vi "Hardware - NI 9751-3 (DI Driver) Host.vi"() -> ()   [LabVIEW 2015, in "ECS-Host.lvlib"]
uses:
  ECS-Host.lvlib
  <vilib>/addons/Software Calibration Management/XControls/SubHost.xctl
panel:
  in  "DisableOnCrit":bool caption="Disable On Crit?"
  in  "OpenCircuitOverride":bool
  in  "Clear Faults":bool
  out "FPGAReadError":bool
  out "FPGAWriteError":bool
  in  "OneShot":bool
  out "ShortCircuitFault":bool
  out "PSOverloadFault":bool
  out "PSChargeFault":bool
  out "ModuleTempFault":bool
  out "LowVoltageDriverFault":bool
  out "HighVoltageLimitFault":bool
  out "HighVoltageDriverFault":bool
  out "FI3OpenCircuit":bool
  out "FI2OpenCircuit":bool
  out "FI1OpenCircuit":bool
  out "Ch3TimingViolation":bool
  out "Ch3PulseOverlap":bool
  out "Ch2TimingViolation":bool
  out "Ch2PulseOverlap":bool
  out "Ch1TimingViolation":bool
  out "Ch1PulseOverlap":bool
  out "MinOffTimeCAD":sgl caption="[]"
  in  "MinOffTime":sgl caption="[]"
  in  "Ch3Enable":bool
  in  "ModuleEnable":bool
  in  "InjectionEnable":bool
  in  "PowerSupplyEnable":bool
  out "ModulePresent":bool
  in  "Phase1FirstPeakEnable":bool
  in  "PiezoEnable":bool
  in  "PiezoInvert":bool
  in  "OneShotSelect":enum32{"a", "b", "c", "d"}(ring)
  in  "OneShotTime":sgl caption="[msec]" format="%#.3f"
  in  "DI3 Scope":T1(xcontrol)
  in  "_DI3_IPhaseDriveArray":bool[](array[boolean]) caption="IPhaseDriveArray"
  in  "IPhaseDuration":sgl[](array[numeric]) min=0 max=5 step=0.001 format="%#.3g"
  in  "IPhaseCurrentLower":sgl[](array[numeric]) min=0 max=30 step=0.1 format="%#.3g"
  in  "IPhaseCurrentUpper":sgl[](array[numeric]) min=0 max=30 step=0.1 format="%#.3g"
  out "BatteryVoltage":sgl=21.08 caption="Battery Voltage"
  out "InternalHighVoltage":sgl=100.0 caption="Internal High Voltage" max=100
  out "ExternalHighVoltage":sgl caption="External High Voltage"
  out "_OLIntegrator_Display":sgl caption="Overload Integrator" format="%#.1g"
  out "ModuleTemperature":sgl=21.08 caption="Module Temp"
  in  "BackBoostTime":sgl caption="[msec]" min=0 max=0.4 step=0.01 format="%#.3f"
  in  "HighVTarget":sgl caption="[V]" max=100 format="%#.1f"
  out "ModuleRev":string
  in  "Ch2Enable":bool
  in  "Ch1Enable":bool
  out "OLIntegrator":u32 caption="Overload Integrator"
  in  "IPhaseDrive":u8
  # "[C]"
  # "Module Temp"
  # "Battery Voltage"
  # "[V]"
  # "Internal High Voltage"
  # "[V]"
  # "External High Voltage"
  # "[V]"
  # "Overload Integrator"
  # "[%]"
  # "[Amps]"
  # "[Amps]"
  # "[ms]"
  # "1"
  # "2"
  # "3"
  # "4"
  # "5"
  # "6"
  # "7"
  # "8"
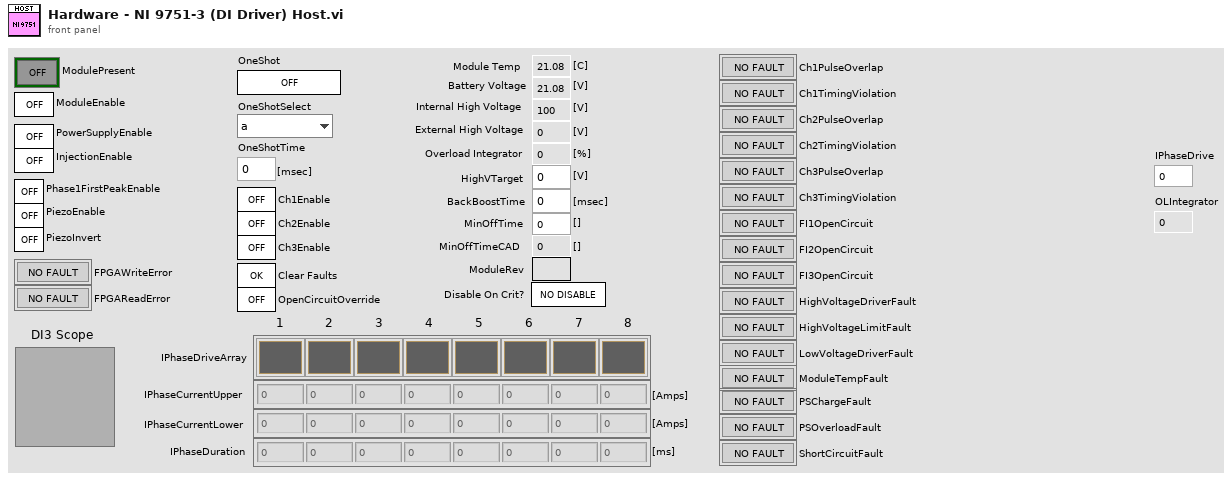
[diagram p1: front panel]
types:
  T1 = cluster{"Name":string, "Host VI":path, "Pairing File":path, "Display Name":string}
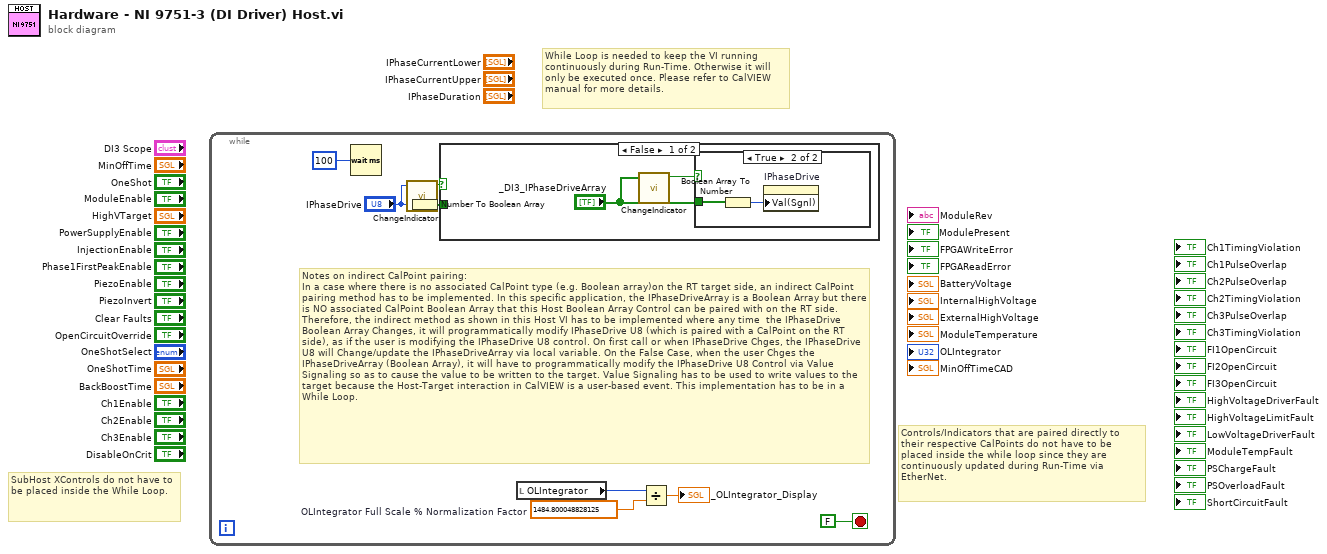
[diagram p0: block diagram]
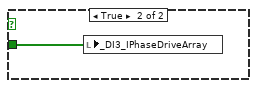
[diagram p3: hidden frame]
diagram:
  # "Controls/Indicators that are paired directly to their respective CalPoints do not have to be placed inside the while loop since they are continuously updated during Run-Time via EtherNet."
  # "SubHost XControls do not have to be placed inside the While Loop."
  # "While Loop is needed to keep the VI running\ncontinuously during Run-Time. Otherwise it will only be executed once. Please refer to CalVIEW manual for more details."
  n1 = while {
    stop <- FALSE stop-if-true
    w2 = sgl 1484.8  # OLIntegrator Full Scale % Normalization Factor
    # "Notes on indirect CalPoint pairing:\nIn a case where there is no associated CalPoint type (e.g. Boolean array)on the RT target side, an indirect CalPoint pairing method has to be implemented. In this specific application, the IPhaseDriveArray is a Boolean Array but there is NO associated CalPoint Boolean Array that this Host Boolean Array Control can be paired with on the RT side. Therefore, the indirect method as shown in this Host VI has to be implemented where any time  the IPhaseDrive Boolean Array Changes, it will programmatically modify IPhaseDrive U8 (which is paired with a CalPoint on the RT side), as if the user is modifying the IPhaseDrive U8 control. On first call or when IPhaseDrive Chges, the IPhaseDrive U8 will Change/update the IPhaseDriveArray via local variable. On the False Case, when the user Chges the IPhaseDriveArray (Boolean Array), it will have to programmatically modify the IPhaseDrive U8 Control via Value Signaling so as to cause the value to be written to the target. Value Signaling has to be used to write values to the target because the Host-Target interaction in CalVIEW is a user-based event. This implementation has to be in a While Loop."
    n2 = Wait (ms)(milliseconds to wait=u32 100) -> ()  [unwired: 1 out]
    n3 = call "ChangeIndicator.vi"("Input"="IPhaseDrive") -> ("Change"=w5:bool)  [unwired: 9 in]
    n4 = Number To Boolean Array(number="IPhaseDrive") -> (Boolean array=w6:bool[])
    n5 = case shown="False" w5 {
      tunnel: w6 -> [_ w13]
      frame False {
        n6 = call "ChangeIndicator.vi"("Input"="_DI3_IPhaseDriveArray") -> ("Change"=w9:bool)  [unwired: 9 in]
        n7 = case shown="True" w9 {
          tunnel: "_DI3_IPhaseDriveArray" -> [_ w11]
          frame False {
          }
          frame True {
            n8 = Boolean Array To Number(Boolean array=w11) -> (number=w12:u8)
            n9 = property on="IPhaseDrive" class="DigNum (strict)"("Val(Sgnl)"=w12) -> ()  [unwired: 2 in, 2 out]
          }
        }
      }
      frame True {
        n10 = local write "_DI3_IPhaseDriveArray"(w13) -> ()
      }
    }
    n11 = local read "OLIntegrator"() -> (w3:u32)
    n12 = Divide(x=w3, y=w2) -> (x/y=→"_OLIntegrator_Display":sgl)
  }
